vi "ScaleandControl.vi"(1 "button info":T2, 2 "axis info":T1) -> (0 "String":string)   [LabVIEW 2010]
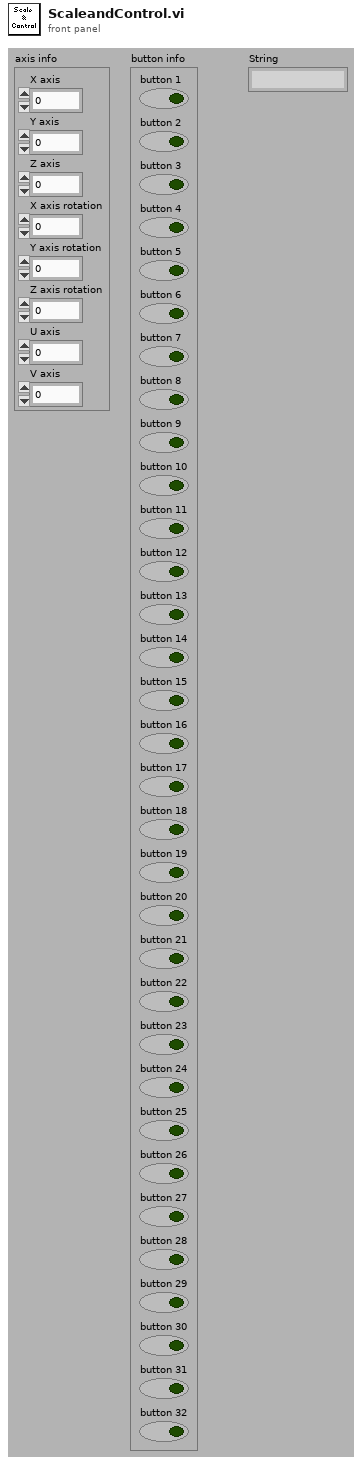
[diagram p1: front panel]
types:
  T1 = cluster{"X axis":i32, "Y axis":i32, "Z axis":i32, "X axis rotation":i32, "Y axis rotation":i32, "Z axis rotation":i32, "U axis":i32, "V axis":i32}
  T2 = cluster{"button 1":bool, "button 2":bool, "button 3":bool, "button 4":bool, "button 5":bool, "button 6":bool, "button 7":bool, "button 8":bool, "button 9":bool, "button 10":bool, "button 11":bool, "button 12":bool, "button 13":bool, "button 14":bool, "button 15":bool, "button 16":bool, "button 17":bool, "button 18":bool, "button 19":bool, "button 20":bool, "button 21":bool, "button 22":bool, "button 23":bool, "button 24":bool, "button 25":bool, "button 26":bool, "button 27":bool, "button 28":bool, "button 29":bool, "button 30":bool, "button 31":bool, "button 32":bool}
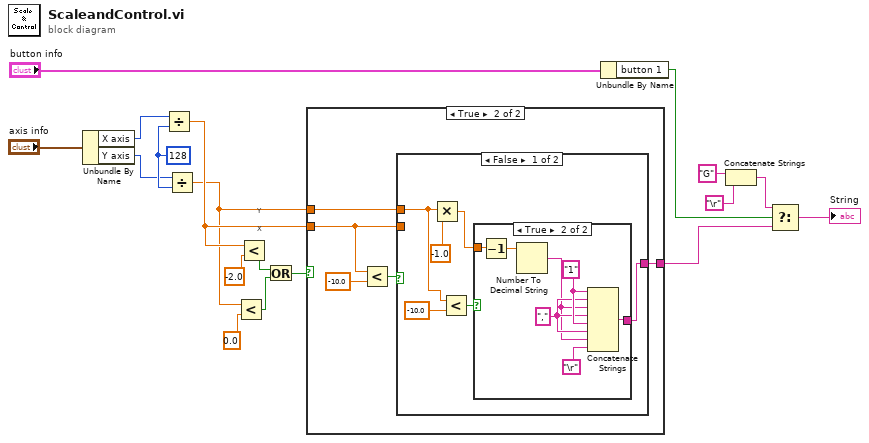
[diagram p0: block diagram]
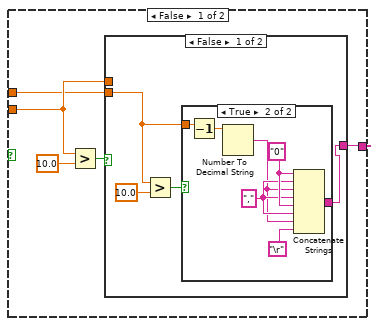
[diagram p2: hidden frame]
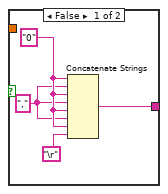
[diagram p3: hidden frame]
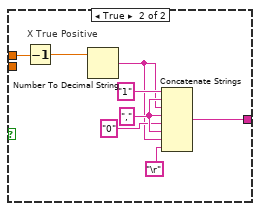
[diagram p4: hidden frame]
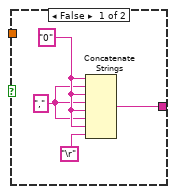
[diagram p5: hidden frame]
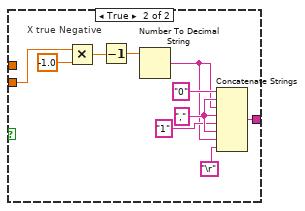
[diagram p6: hidden frame]
diagram:
  w6 = 128 ("y")
  # "X"
  # "Y"
  n1 = Unbundle By Name("axis info") -> ("X axis"=w4:i32, "Y axis"=w3:i32)
  n2 = Divide(x=w4, y=w6) -> (x/y=w9:dbl)
  n3 = Divide(x=w3, y=w6) -> (x/y=w2:dbl)
  n4 = Less?(x=w2, y=0.0) -> (x < y?=w8:bool)
  n5 = Less?(x=w9, y=-2.0) -> (x < y?=w11:bool)
  n6 = Or(x=w11, y=w8) -> (x .or. y?=w7:bool)
  n7 = case shown="True" w7 {
    tunnel: [w21 w49] -> w16
    tunnel: w9 -> [w20 w48]
    tunnel: w2 -> [w19 w47]
    frame False {
      n8 = Greater?(x=w20, y=10.0) -> (0:w23:bool)
      n9 = case shown="False" w23 {
        tunnel: [w25 w44] -> w21
        tunnel: w20 -> [_ w40]
        tunnel: w19 -> [w24 _]
        frame False {
          n10 = Greater?(x=w24, y=10.0) -> (0:w26:bool)
          n11 = case shown="True" w26 {
            tunnel: [w28 w35] -> w25
            tunnel: w24 -> [_ w33]
            frame False {
              w29 = "," ("string")
              w31 = "0" ("string")
              n12 = Concatenate Strings(w31, w29, w31, w29, w31, w29, w31, "\r") -> (w28:string)
            }
            frame True {
              w36 = "," ("string")
              w38 = "0" ("string")
              n13 = Decrement(x=w33) -> (x-1=w32:dbl)
              n14 = Number To Decimal String(number=w32) -> (decimal integer string=w34:string)  [unwired: 1 in]
              n15 = Concatenate Strings(w38, w36, w34, w36, w38, w36, w34, "\r") -> (w35:string)
            }
          }
        }
        frame True {
          w46 = "," ("string")
          # "X True Positive"
          n16 = Decrement(x=w40) -> (x-1=w39:dbl)
          n17 = Number To Decimal String(number=w39) -> (decimal integer string=w41:string)  [unwired: 1 in]
          n18 = Concatenate Strings("1" ("string"), w46, w41, w46, "0" ("string"), w46, w41, "\r") -> (w44:string)
        }
      }
    }
    frame True {
      n19 = Less?(x=w48, y=-10.0) -> (x < y?=w51:bool)
      n20 = case shown="False" w51 {
        tunnel: [w55 w75] -> w49
        tunnel: w48 -> [_ w71]
        tunnel: w47 -> [w52 _]
        frame False {
          n21 = Multiply(x=w52, y=-1.0) -> (x*y=w53:dbl)
          n22 = Less?(x=w52, y=-10.0) -> (x < y?=w56:bool)
          n23 = case shown="True" w56 {
            tunnel: [w58 w65] -> w55
            tunnel: w53 -> [_ w63]
            frame False {
              w59 = "," ("string")
              w61 = "0" ("string")
              n24 = Concatenate Strings(w61, w59, w61, w59, w61, w59, w61, "\r") -> (w58:string)
            }
            frame True {
              w66 = "," ("string")
              w68 = "1" ("string")
              n25 = Decrement(x=w63) -> (x-1=w62:dbl)
              n26 = Number To Decimal String(number=w62) -> (decimal integer string=w64:string)  [unwired: 1 in]
              n27 = Concatenate Strings(w68, w66, w64, w66, w68, w66, w64, "\r") -> (w65:string)
            }
          }
        }
        frame True {
          w78 = "," ("string")
          # "X true Negative"
          n28 = Multiply(x=w71, y=-1.0) -> (x*y=w70:dbl)
          n29 = Decrement(x=w70) -> (x-1=w69:dbl)
          n30 = Number To Decimal String(number=w69) -> (decimal integer string=w72:string)  [unwired: 1 in]
          n31 = Concatenate Strings("0" ("string"), w78, w72, w78, "1" ("string"), w78, w72, "\r") -> (w75:string)
        }
      }
    }
  }
  n32 = Unbundle By Name("button info") -> ("button 1"=w17:bool)
  n33 = Concatenate Strings("G" ("string"), "\r") -> (w15:string)
  n34 = Select(t=w15, s=w17, f=w16) -> (s? t:f=→"String":string)
